vi "ifr2025 Initialize.vi"(8 "error in (no error)":errorcluster {"code" format="%.0x"}, 9 "reset device (Reset Device)":bool, 10 "id query (Do Query)":bool=TRUE, 11 "resource name":refnum<visa-resource-name>="visa://marconi/GPIB0::6::INSTR") -> (0 "error out":errorcluster {"code" format="%.0x"}, 3 "instrument handle out":refnum<visa-resource-name>)   [LabVIEW 2009]
doc: "This function must be called to open a VISA session to an instrument."
uses:
  Ifr2025_32.dll
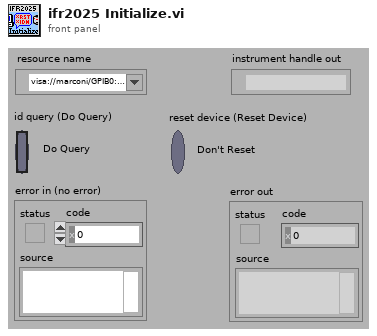
[diagram p1: front panel]
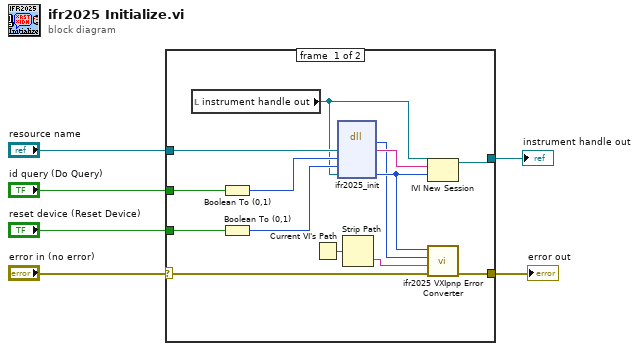
[diagram p0: block diagram]
diagram:
  n1 = case shown="No Error" "error in (no error)" {
    selector: "error in (no error)" -> [w8 w21]
    tunnel: [w7 w21] -> w5
    tunnel: "resource name" -> [w16 _]
    tunnel: [w15 _] -> w3
    tunnel: "id query (Do Query)" -> [w13 _]
    tunnel: "reset device (Reset Device)" -> [w12 _]
    frame #0 {
      n2 = local read "instrument handle out"() -> (w14:refnum<visa-resource-name>)
      n3 = Boolean To (0,1)(Boolean=w13) -> (0, 1=w20:i16)
      n4 = Boolean To (0,1)(Boolean=w12) -> (0, 1=w19:i16)
      n5 = Current VI's Path() -> (path=w17:path)
      n6 = dll-call lib="P:/inst/Marconi 2024 Signal Generator/source/labview/ifr2025/ifr2025/ifr2025_*.*" fn="ifr2025_init"("resource name"=w16, "id query"=w20, "reset device"=w19, "instrument handle"=w14) -> ("status"=w10:i32, "resource name"=w18:string, "instrument handle"=w11:u32)  [unwired: 5 in, 2 out]
      n7 = Strip Path(path=w17) -> (name=w9:string)  [unwired: 1 out]
      n8 = IVI New Session(9:w11, 10:w18, 11:w14) -> (3:w15:refnum<visa-resource-name>)
      n9 = call "ifr2025 VXIpnp Error Converter.vi"("error in (no error)"=w8, "name of VI (\"\")"=w9, "CVI error code (0)"=w10, "instrument handle"=w11) -> ("error out"=w7:errorcluster)  [unwired: 7 out]
    }
    frame #1 {
    }
  }
  "error out" <- w5
  "instrument handle out" <- w3
